vi "Various File Format Saver.vi"(8 "Incoming Data to be Saved":dbl[][](array[numeric]), 9 "File Name":string, 10 "File Format":T1(radio), 11 "Folder to Save Data":path) -> ()   [LabVIEW 2020]
doc: "Allows the user to save their file in various formats.\n\nArgs:\nFile Format: The desired format from the user ranging from ASCII, CSV and .MAT file\nFolder to Save Data: Folder that the data needs to be saved in\nFile Name: Name of the file that is being created\nIncoming Data to be Saved: Data from the oscilloscope or sample data for demonstration purposes"
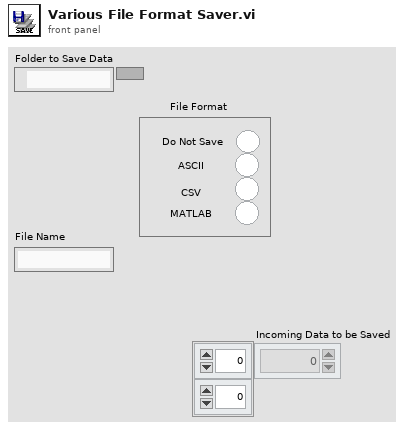
[diagram p1: front panel]
types:
  T1 = enum32{"No Selection", "Do Not Save", "ASCII", "CSV", "MATLAB"}
  T2 = enum16{"open", "replace", "create", "open or create", "replace or create", "replace or create with confirmation"}
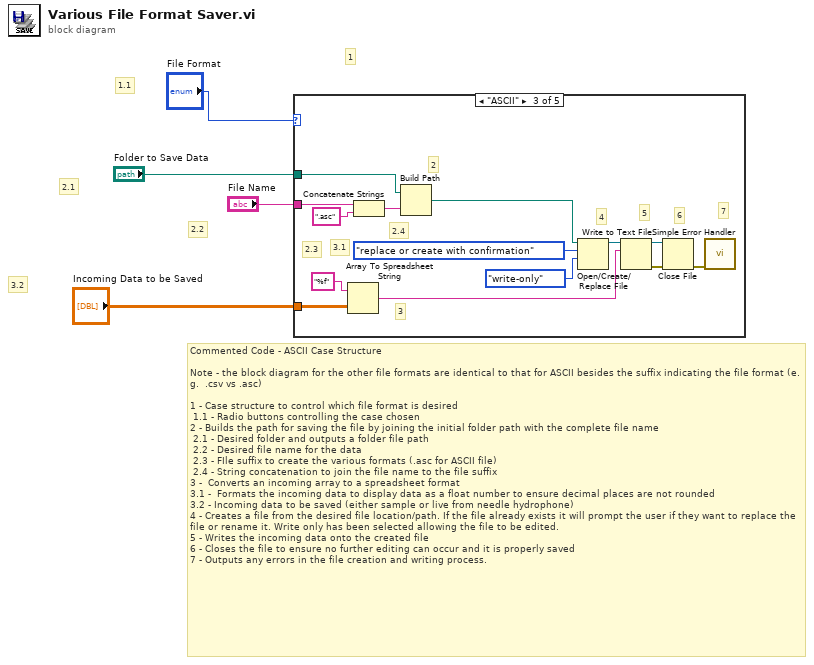
[diagram p0: block diagram]
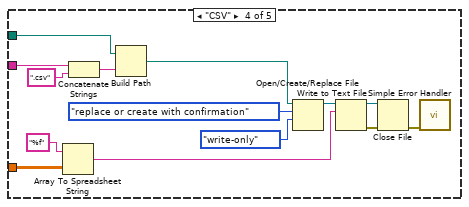
[diagram p4: hidden frame]
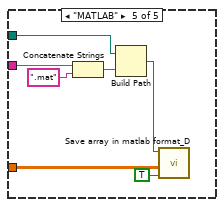
[diagram p5: hidden frame]
diagram:
  # "3.2"
  # "2.2"
  # "2.1"
  # "1.1"
  # "1"
  # "Commented Code - ASCII Case Structure\n\nNote - the block diagram for the other file formats are identical to that for ASCII besides the suffix indicating the file format (e.g.  .csv vs .asc)\n\n1 - Case structure to control which file format is desired \n 1.1 - Radio buttons controlling the case chosen\n2 - Builds the path for saving the file by joining the initial folder path with the complete file name\n 2.1 - Desired folder and outputs a folder file path\n 2.2 - Desired file name for the data\n 2.3 - FIle suffix to create the various formats (.asc for ASCII file)\n 2.4 - String concatenation to join the file name to the file suffix\n3 -  Converts an incoming array to a spreadsheet format\n3.1 -  Formats the incoming data to display data as a float number to ensure decimal places are not rounded\n3.2 - Incoming data to be saved (either sample or live from needle hydrophone) \n4 - Creates a file from the desired file location/path. If the file already exists it will prompt the user if they want to replace the file or rename it. Write only has been selected allowing the file to be edited.\n5 - Writes the incoming data onto the created file\n6 - Closes the file to ensure no further editing can occur and it is properly saved\n7 - Outputs any errors in the file creation and writing process."
  n1 = case shown="\"ASCII\"" "File Format" {
    tunnel: "Incoming Data to be Saved" -> [_ _ w5 w21 w34]
    tunnel: "Folder to Save Data" -> [_ _ w7 w20 w36]
    tunnel: "File Name" -> [_ _ w6 w19 w35]
    frame "No Selection" {
    }
    frame "Do Not Save" {
    }
    frame "ASCII" {
      # "2.4"
      # "2.3"
      # "7"
      # "6"
      # "5"
      # "4"
      # "3.1"
      # "3"
      # "2"
      n2 = Array To Spreadsheet String(array=w5, 3:"%f" ("format string")) -> (spreadsheet string=w17:string)  [unwired: 1 in]
      n3 = Concatenate Strings(w6, ".asc" ("string")) -> (w12:string)
      n4 = Build Path(base path=w7, name or relative path=w12) -> (appended path=w13:path)
      n5 = Open/Create/Replace File(file path (use dialog)=w13, operation (0:open)=T2."replace or create with confirmation", access (0:read/write)=enum16{"read/write", "read-only", "write-only"}."write-only") -> (refnum out=w18:refnum<file>)  [unwired: 1 in, 4 out]
      n6 = Write to Text File(file (use dialog)=w18, text=w17) -> (refnum out=w16:refnum<file>, error out=w15:errorcluster)  [unwired: 2 in, 1 out]
      n7 = Close File(refnum=w16, error in=w15) -> (error out=w14:errorcluster)  [unwired: 1 out]
      n8 = call <vilib>:"Simple Error Handler.vi"("error in (no error)"=w14) -> ()  [unwired: 1 in, 8 out]
    }
    frame "CSV" {
      n9 = Array To Spreadsheet String(array=w21, 3:"%f" ("format string")) -> (spreadsheet string=w28:string)  [unwired: 1 in]
      n10 = Concatenate Strings(w19, ".csv" ("string")) -> (w27:string)
      n11 = Build Path(base path=w20, name or relative path=w27) -> (appended path=w26:path)
      n12 = Open/Create/Replace File(file path (use dialog)=w26, operation (0:open)=T2."replace or create with confirmation", access (0:read/write)=enum16{"read/write", "read-only", "write-only"}."write-only") -> (refnum out=w32:refnum<file>)  [unwired: 1 in, 4 out]
      n13 = Write to Text File(file (use dialog)=w32, text=w28) -> (refnum out=w29:refnum<file>, error out=w30:errorcluster)  [unwired: 2 in, 1 out]
      n14 = Close File(refnum=w29, error in=w30) -> (error out=w31:errorcluster)  [unwired: 1 out]
      n15 = call <vilib>:"Simple Error Handler.vi"("error in (no error)"=w31) -> ()  [unwired: 1 in, 8 out]
    }
    frame "MATLAB" {
      n16 = Concatenate Strings(w35, ".mat" ("string")) -> (w38:string)
      n17 = Build Path(base path=w36, name or relative path=w38) -> (appended path=w39:path)
      n18 = call "Save array in matlab format_D"("append to file? (new file:F)"=TRUE, "2D array"=w34, "file path (dialog if empty)"=w39) -> ()  [unwired: 4 in, 1 out]
    }
  }
